vi "Inpsig.vi"(1 "Множитель":dbl=10.0) -> (0 "Случайное число":dbl)   [LabVIEW 2011]
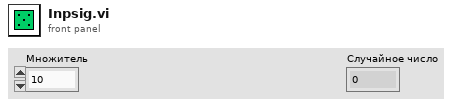
[diagram p1: front panel]
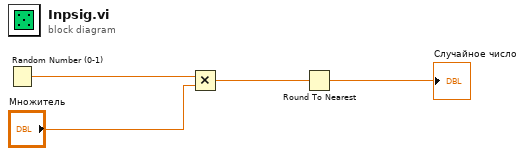
[diagram p0: block diagram]
diagram:
  n1 = Random Number (0-1)() -> (number: 0 to 1=w2:dbl)
  n2 = Multiply(x=w2, y="Множитель") -> (x*y=w4:dbl)
  n3 = Round To Nearest(number=w4) -> (nearest integer value=→"Случайное число":dbl)
